vi "Event Last Ack.vi"(10 "Event jettl":refnum<class "Event jettl.lvclass">, 11 "Base Queue jettl in":refnum<class "Base Queue jettl.lvclass">) -> (3 "Base Queue jettl out":refnum<class "Base Queue jettl.lvclass">)   [LabVIEW 2021, in "jettl.lvlib" / "Base Queue jettl.lvlib" / "Base Queue jettl.lvclass"]
uses:
  Base Queue jettl.lvclass
  Event jettl/Event jettl.lvclass
  Base Queue jettl.lvclass/Base Queue jettl.ctl
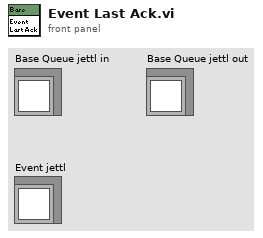
[diagram p1: front panel]
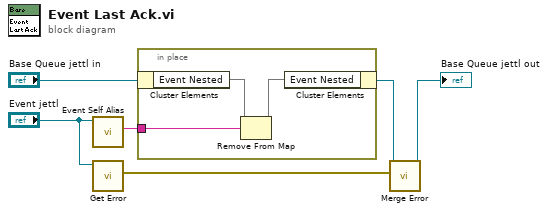
[diagram p0: block diagram]
diagram:
  n1 = call-dynamic "Event Self Alias.vi"("jettl in"="Event jettl") -> ("Event Self Alias"=w1:string)  [unwired: 10 in]
  n2 = call-dynamic "Get Error.vi"("jettl in"="Event jettl") -> ("Error"=w6:errorcluster)  [unwired: 10 in]
  n3 = in-place {
    in-place-border: w1 -> [w7]
    n4 = in-place-cluster #1("Base Queue jettl in") -> ("Event Nested"=w8:map{string, refnum<data-value>})
    n5 = Remove From Map(10:w7, 11:w8) -> (3:w9:map{string, refnum<data-value>})  [unwired: 2 out]
    n6 = in-place-cluster #1("Event Nested"=w9) -> (w5:refnum<class "Base Queue jettl.lvclass">)
  }
  n7 = call-dynamic "Merge Error.vi"("Error"=w6, "Base Queue jettl in"=w5) -> ("Base Queue jettl out"=→"Base Queue jettl out":refnum<class "Base Queue jettl.lvclass">)  [unwired: 9 in]
